vi "LogFFT with WIndowing.vi"(5 "FFT Pad?":bool, 6 "window":T1=2 items=["Rectangle"=0, "Hanning"=1, "Hamming"=2, "Blackman-Harris"=3, "Exact Blackman"=4, "Blackman"=5, "Flat Top"=6, "4 Term B-Harris "=7, "7 Term B-Harris"=8, "Low Sidelobe"=9, "Blackman Nuttall"=11, "Triangle"=30, "Bartlett-Hanning"=31, "Bohman"=32, "Parzen"=33, "Welch"=34, "Kaiser"=60, "Dolph-Chebyshev"=61, "Gaussian"=62], 7 "Window":bool, 9 "Padded FT Size":i32, 10 "FFT {X}":cdb[](array[numeric])) -> (2 "Log{Mag(FFT)}":dbl[](array[numeric]))   [LabVIEW 2012]
uses:
  <vilib>/Analysis/4window.llb/windowTd.ctl
  <vilib>/Analysis/0measdsp.llb/Scaled Time Domain Window (CDB).vi
  <vilib>/Analysis/2dsp.llb/Inverse Complex FFT.vi
  <vilib>/Analysis/NI_AALPro.lvlib
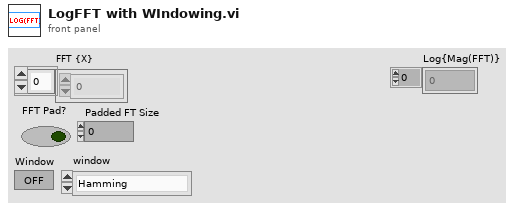
[diagram p1: front panel]
types:
  T1 = typedef "NI_AALPro.lvlib/windowTd.ctl" = u32
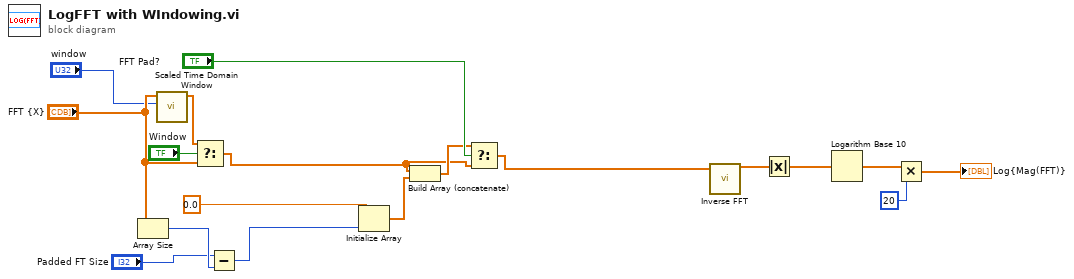
[diagram p0: block diagram]
diagram:
  n1 = Array Size(array="FFT {X}") -> (size(s)=w10:i32)
  n2 = call-poly <vilib>:"Scaled Time Domain Window.vi"("window"="window", "X"="FFT {X}") -> ("Windowed X"=w4:cdb[])  [unwired: 7 in, 2 out]
  n3 = Select(t=w4, s="Window", f="FFT {X}") -> (s? t:f=w3:cdb[])
  n4 = Subtract(x="Padded FT Size", y=w10) -> (x-y=w8:i32)
  n5 = Initialize Array(0.0 ("element"), w8) -> (w13:dbl[])
  n6 = Build Array (concatenate)(w3, w13) -> (w11:cdb[])
  n7 = Select(t=w11, s="FFT Pad?", f=w3) -> (s? t:f=w1:cdb[])
  n8 = call-poly <vilib>:"Inverse FFT.vi"("FFT {X}"=w1) -> ("X"=w7:cdb[])  [unwired: 9 in, 1 out]
  n9 = Absolute Value(x=w7) -> (abs(x)=w15:dbl[])
  n10 = Logarithm Base 10(1:w15) -> (0:w18:dbl[])
  n11 = Multiply(x=w18, y=20) -> (x*y=→"Log{Mag(FFT)}":dbl[])
